vi "Set Temperature.vi"(8 "error in (no error)":errorcluster, 10 "Setpoint":dbl, 11 "Huber Settings In":T1) -> (0 "error out":errorcluster, 1 "Connection Error":bool, 3 "Huber Settings Out":T1)   [LabVIEW 2018, in "Huber Unistat 410 TCU.lvlib"]
uses:
  Huber Unistat 410 TCU.lvlib
  Huber Unistat 410 Settings.ctl
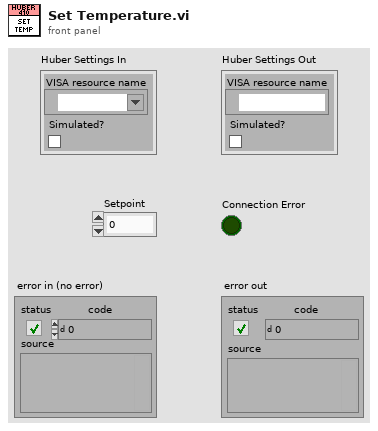
[diagram p1: front panel]
types:
  T1 = typedef "Huber Unistat 410 TCU.lvlib/Huber Unistat 410 Settings.ctl" = cluster{"VISA resource name":refnum<visa-resource-name>, "Simulated?":bool}
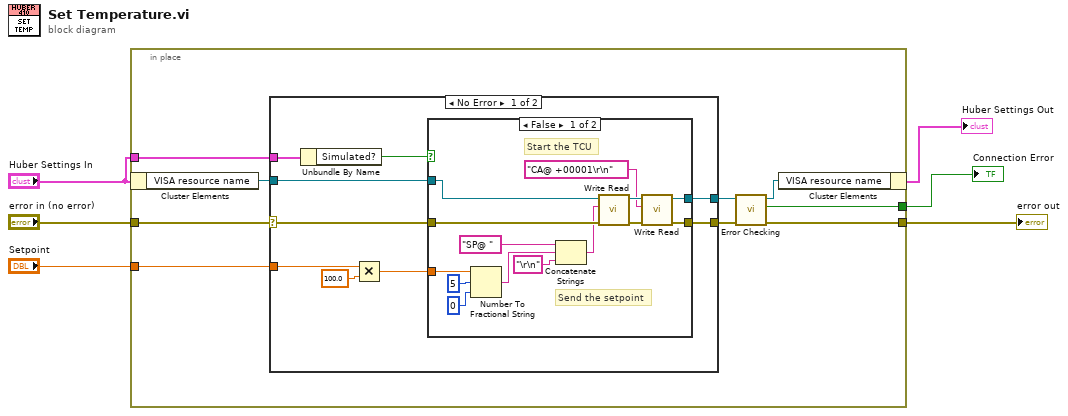
[diagram p0: block diagram]
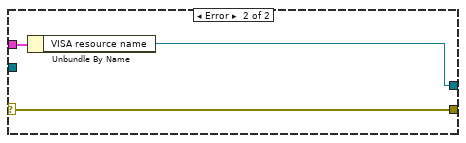
[diagram p3: hidden frame]
diagram:
  n1 = in-place {
    in-place-border: "error in (no error)" -> [w15]
    in-place-border: [w12] -> w5
    in-place-border: "Huber Settings In" -> [w11]
    in-place-border: [w10] -> w4
    in-place-border: "Setpoint" -> [w9]
    n2 = in-place-cluster #1("Huber Settings In") -> ("VISA resource name"=w8:refnum<visa-resource-name>)
    n3 = case shown="No Error" w15 {
      selector: w15 -> [w24 w43]
      tunnel: w11 -> [w20 w42]
      tunnel: [w23 w43] -> w13
      tunnel: [w22 w41] -> w14
      tunnel: w9 -> [w17 _]
      tunnel: w8 -> [w16 _]
      frame No Error {
        n4 = Unbundle By Name(w20) -> ("Simulated?"=w21:bool)
        n5 = Multiply(x=w17, y=100.0) -> (x*y=w18:dbl)
        n6 = case shown="False" w21 {
          tunnel: w24 -> [w31 w40]
          tunnel: [w26 w40] -> w23
          tunnel: [w25 w39] -> w22
          tunnel: w16 -> [w32 w39]
          tunnel: w18 -> [w35 _]
          frame False {
            # "Start the TCU"
            # "Send the setpoint"
            n7 = Number To Fractional String(number=w35, width (-)=i16 5, precision (6)=i16 0) -> (F-format string=w38:string)  [unwired: 1 in]
            n8 = Concatenate Strings("SP@ " ("string"), w38, "\r\n" ("string")) -> (w30:string)
            n9 = call "Write Read.vi"("error in (no error)"=w31, "write string"=w30, "VISA Refnum in"=w32) -> ("error out"=w27:errorcluster, "VISA Refnum out"=w29:refnum<visa-resource-name>)  [unwired: 6 in, 1 out]
            n10 = call "Write Read.vi"("error in (no error)"=w27, "write string"="CA@ +00001\r\n", "VISA Refnum in"=w29) -> ("error out"=w26:errorcluster, "VISA Refnum out"=w25:refnum<visa-resource-name>)  [unwired: 6 in, 1 out]
          }
          frame True {
          }
        }
      }
      frame Error {
        n11 = Unbundle By Name(w42) -> ("VISA resource name"=w41:refnum<visa-resource-name>)
      }
    }
    n12 = call "Error Checking.vi"("error in (no error)"=w13, "VISA resource name"=w14) -> ("error out"=w12:errorcluster, "Connection Error"=w10:bool, "VISA resource name"=w7:refnum<visa-resource-name>)  [unwired: 7 in]
    n13 = in-place-cluster #1("VISA resource name"=w7) -> (→"Huber Settings Out":T1)
  }
  "error out" <- w5
  "Connection Error" <- w4
